vi "LoopVI-V4.vi"() -> ()   [LabVIEW 2013]
uses:
  <vilib>/Utility/file.llb/Read From Spreadsheet File (DBL).vi
panel:
  out "min index(es)":i32
  out "min value":dbl
  out "output array":dbl[](array[numeric])
  out "Collimator afstand":dbl
  out "Spleedbreedte":dbl
  out "Alignment correction":dbl
  out "Background coincidence counts":dbl
  out "Core width":dbl
  out "Fermi Angle":dbl
  out "22na source radius":dbl
  out "Fraction core annihilations":dbl
  out "Minimum summed squared residuals":dbl
  in  "Step size":dbl=1.0 format="%#_13g"
  in  "Begin range":dbl=575.0 format="%#_13g"
  in  "Amount of steps":i32=50
  in  "?":dbl=0.1 format="%#_13g"
  in  "Begin range":dbl=0.5 format="%#_13g"
  in  "Amount of steps":i32=10
  in  "Step size":dbl=0.1 format="%#_13g"
  in  "Begin range":dbl=2.5 format="%#_13g"
  in  "Amount of steps":i32=40
  in  "Step size":dbl=0.1 format="%#_13g"
  in  "Begin range":dbl=1.0 format="%#_13g"
  in  "Amount of steps":dbl=10.0 format="%#_13g"
  in  "Step size":dbl=0.1 format="%#_13g"
  in  "Begin range":dbl=4.0 format="%#_13g"
  in  "Amount of steps":i32=5
  in  "Amount of steps":dbl=4.0 format="%#_13g"
  in  "Step size":dbl=0.1 format="%#_13g"
  in  "Amount of steps":i32=20
  in  "Amount of steps":i32=2
  in  "Begin range":dbl=6.5 format="%#_13g"
  in  "Step size":dbl=0.1 format="%#_13g"
  in  "Begin range":dbl=0.01 format="%#_13g"
  in  "Step size":dbl=0.1 format="%#_13g"
  in  "Begin range":dbl=0.15 format="%#_13g"
  in  "Stop Button":bool
  out "Percentage":dbl format="%#_4f"
  in  "file path (dialog if empty)":path
  in  "Load":bool caption="measurement file\n\n         ??. txt"
  out "free gas model":cluster{"Y":dbl[], "Y":dbl[]}[](graph)
  in  "Fermi angle\n   (mrad)":dbl=7.0
  in  "stop 2":bool
  out "core electrons":cluster{"Y":dbl[], "Y":dbl[]}[](graph)
  in  "core width\n   (mrad)":dbl=5.0
  in  "fraction core\nannihilations":dbl=0.2 min=0.0 max=1.0 step=1e-05
  out "ZICHT  functie":cluster{"Y":dbl[], "Y":dbl[]}[](graph)
  in  "spleetbreedte\n      (mm)":dbl=1.0 min=0.1 max=5.0
  in  "collimator afstand\n       (mm)":dbl=500.0 min=100.0 max=1000.0
  in  "stop 4":bool
  out "XY Graph 4":cluster{ext[], "Array out":ext[]}[](graph)
  in  "alignment correction":dbl min=-10.0 max=10.0 step=0.0001
  in  "background \n coincidence counts":dbl min=0.0 max=100.0
  out "Fermi energy (eV)":dbl format="%#_3g"
  in  "22Na source radius (mm)":dbl=0.1 min=1e-05 max=3.0
  in  "1d - Acar":bool caption="2d - Acar or DB"
  out "2d - Acar 2":bool
  out "2d - Acar 3":bool
  out "2d - Acar 4":bool
  out "XY Graph 5":cluster{ext[], "Array out":ext[]}[](graph)
  out "output cluster 2":cluster{ext[], ext[]}
  out "Sum of squared residuals":dbl
  in  "sigma (mrad) 2":dbl
  # "Step size"
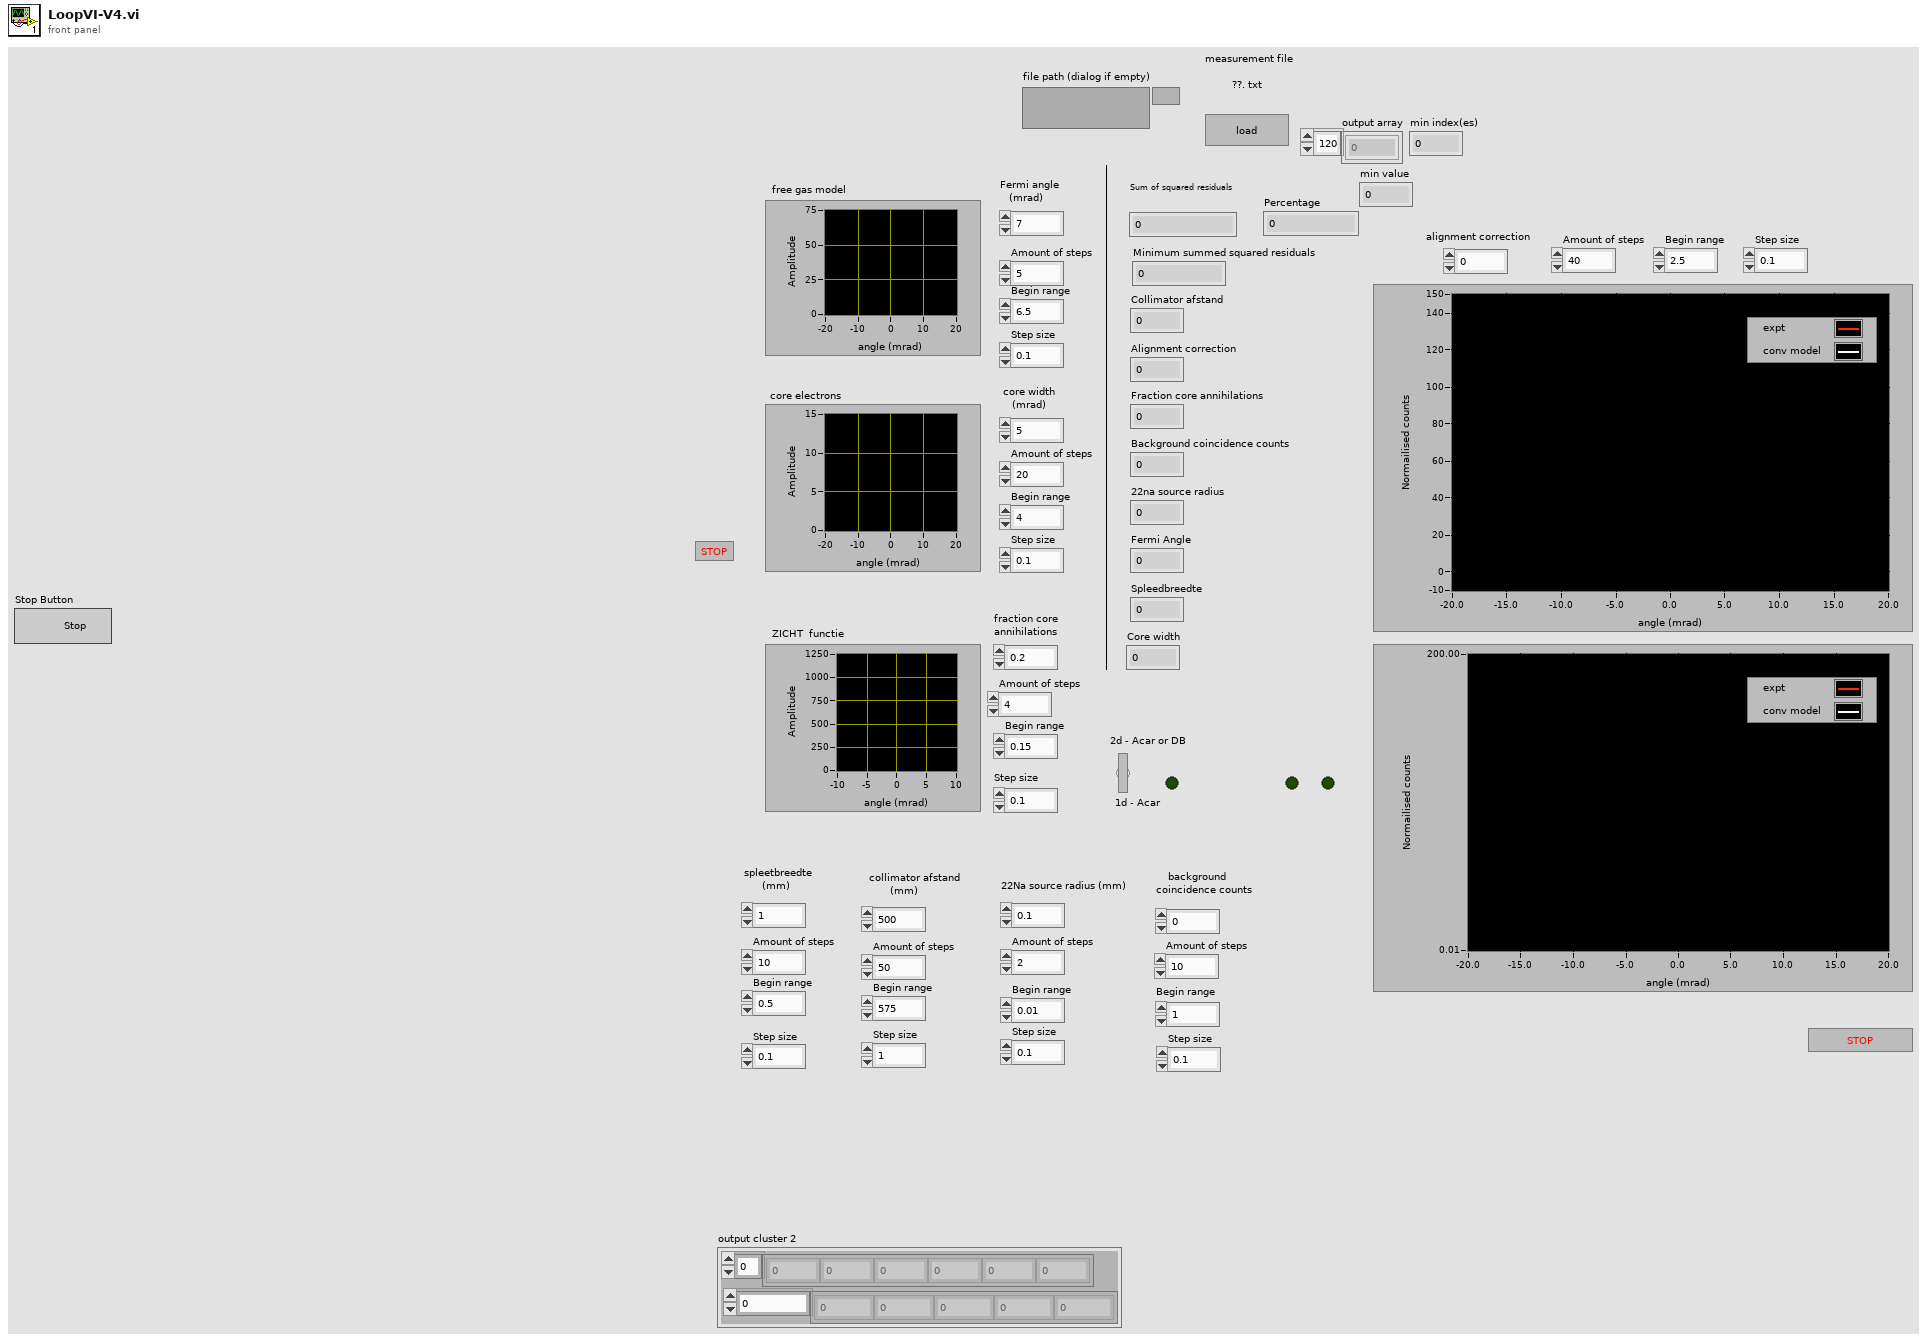
[diagram p1: front panel]
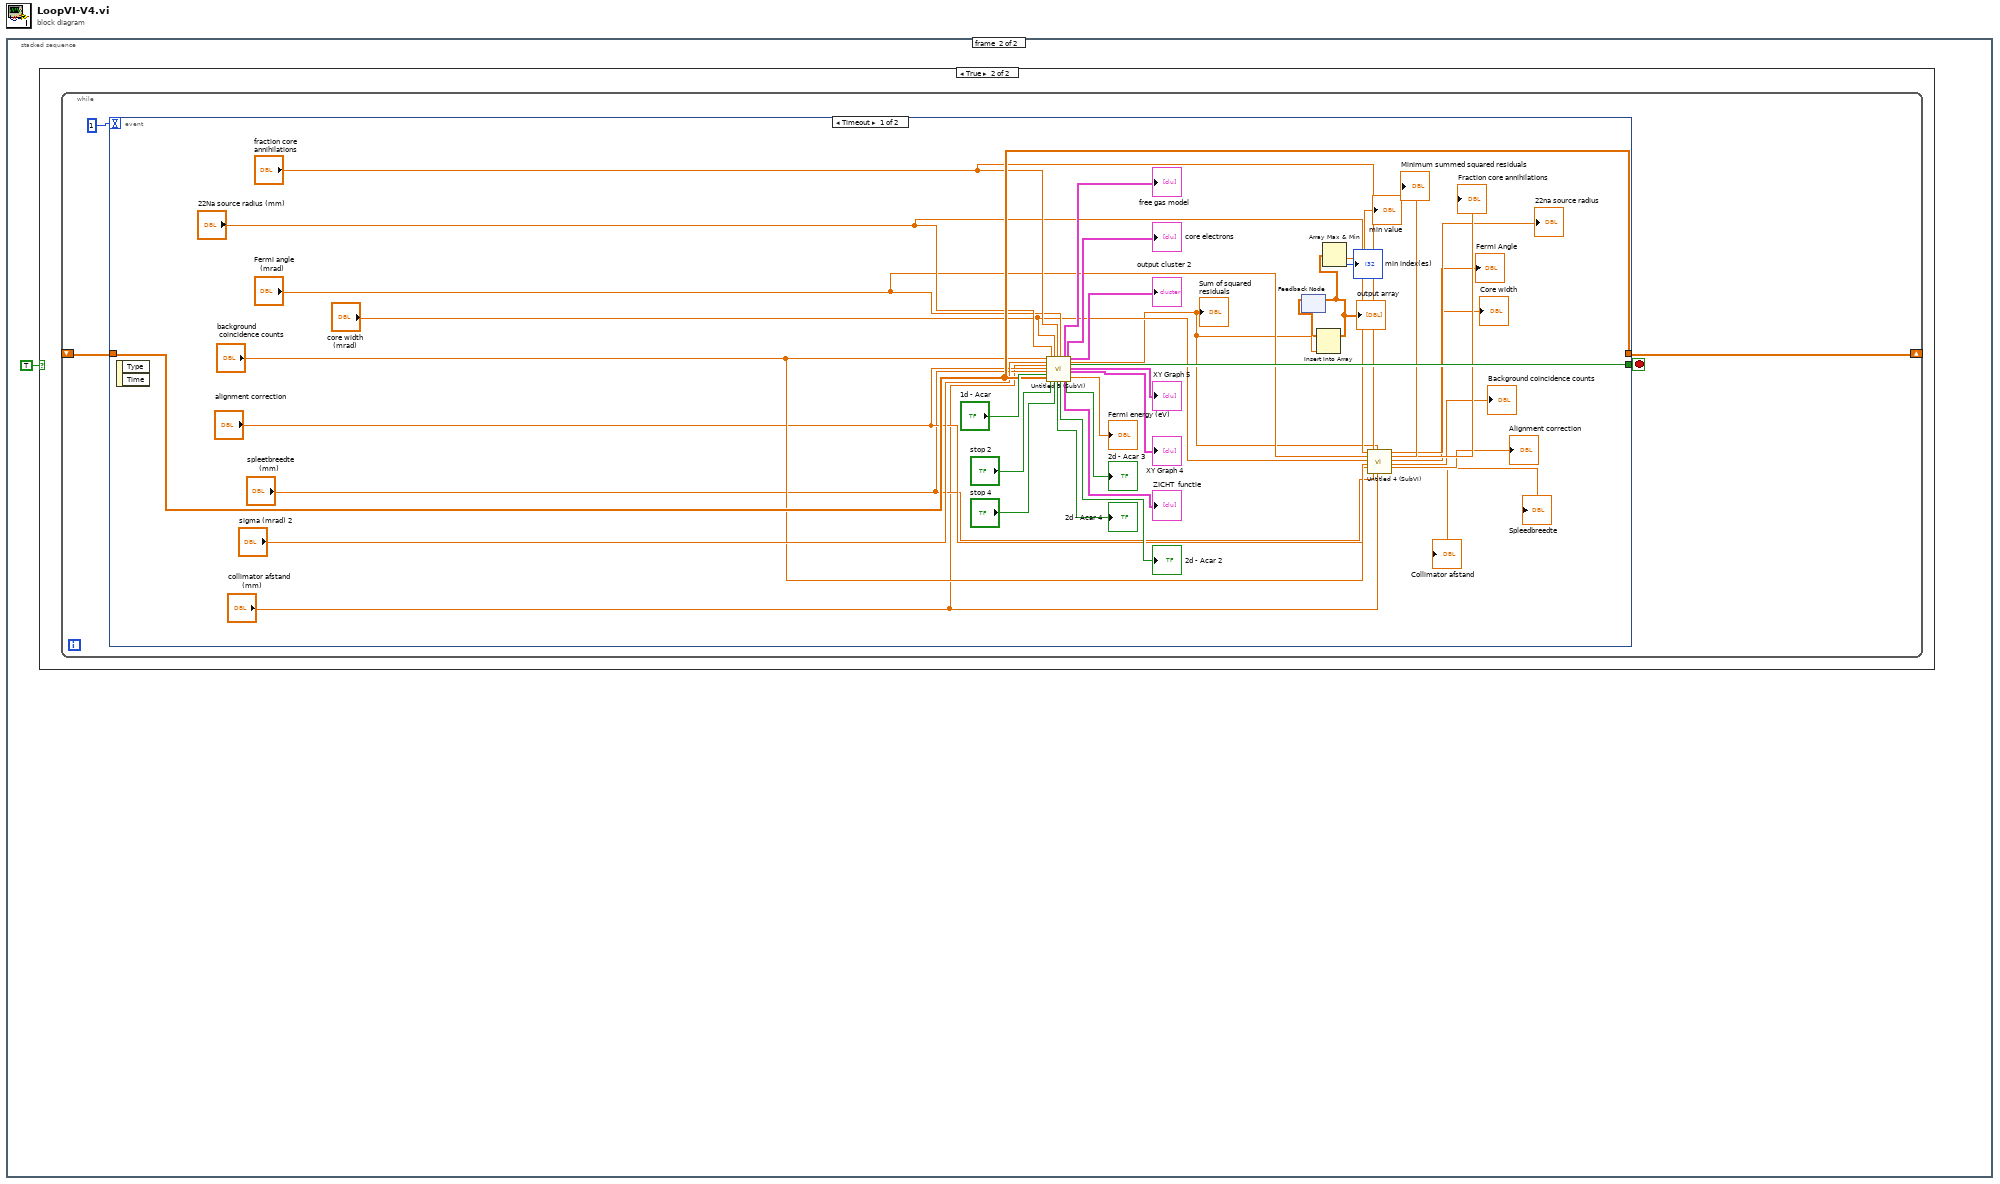
[diagram p0: block diagram]
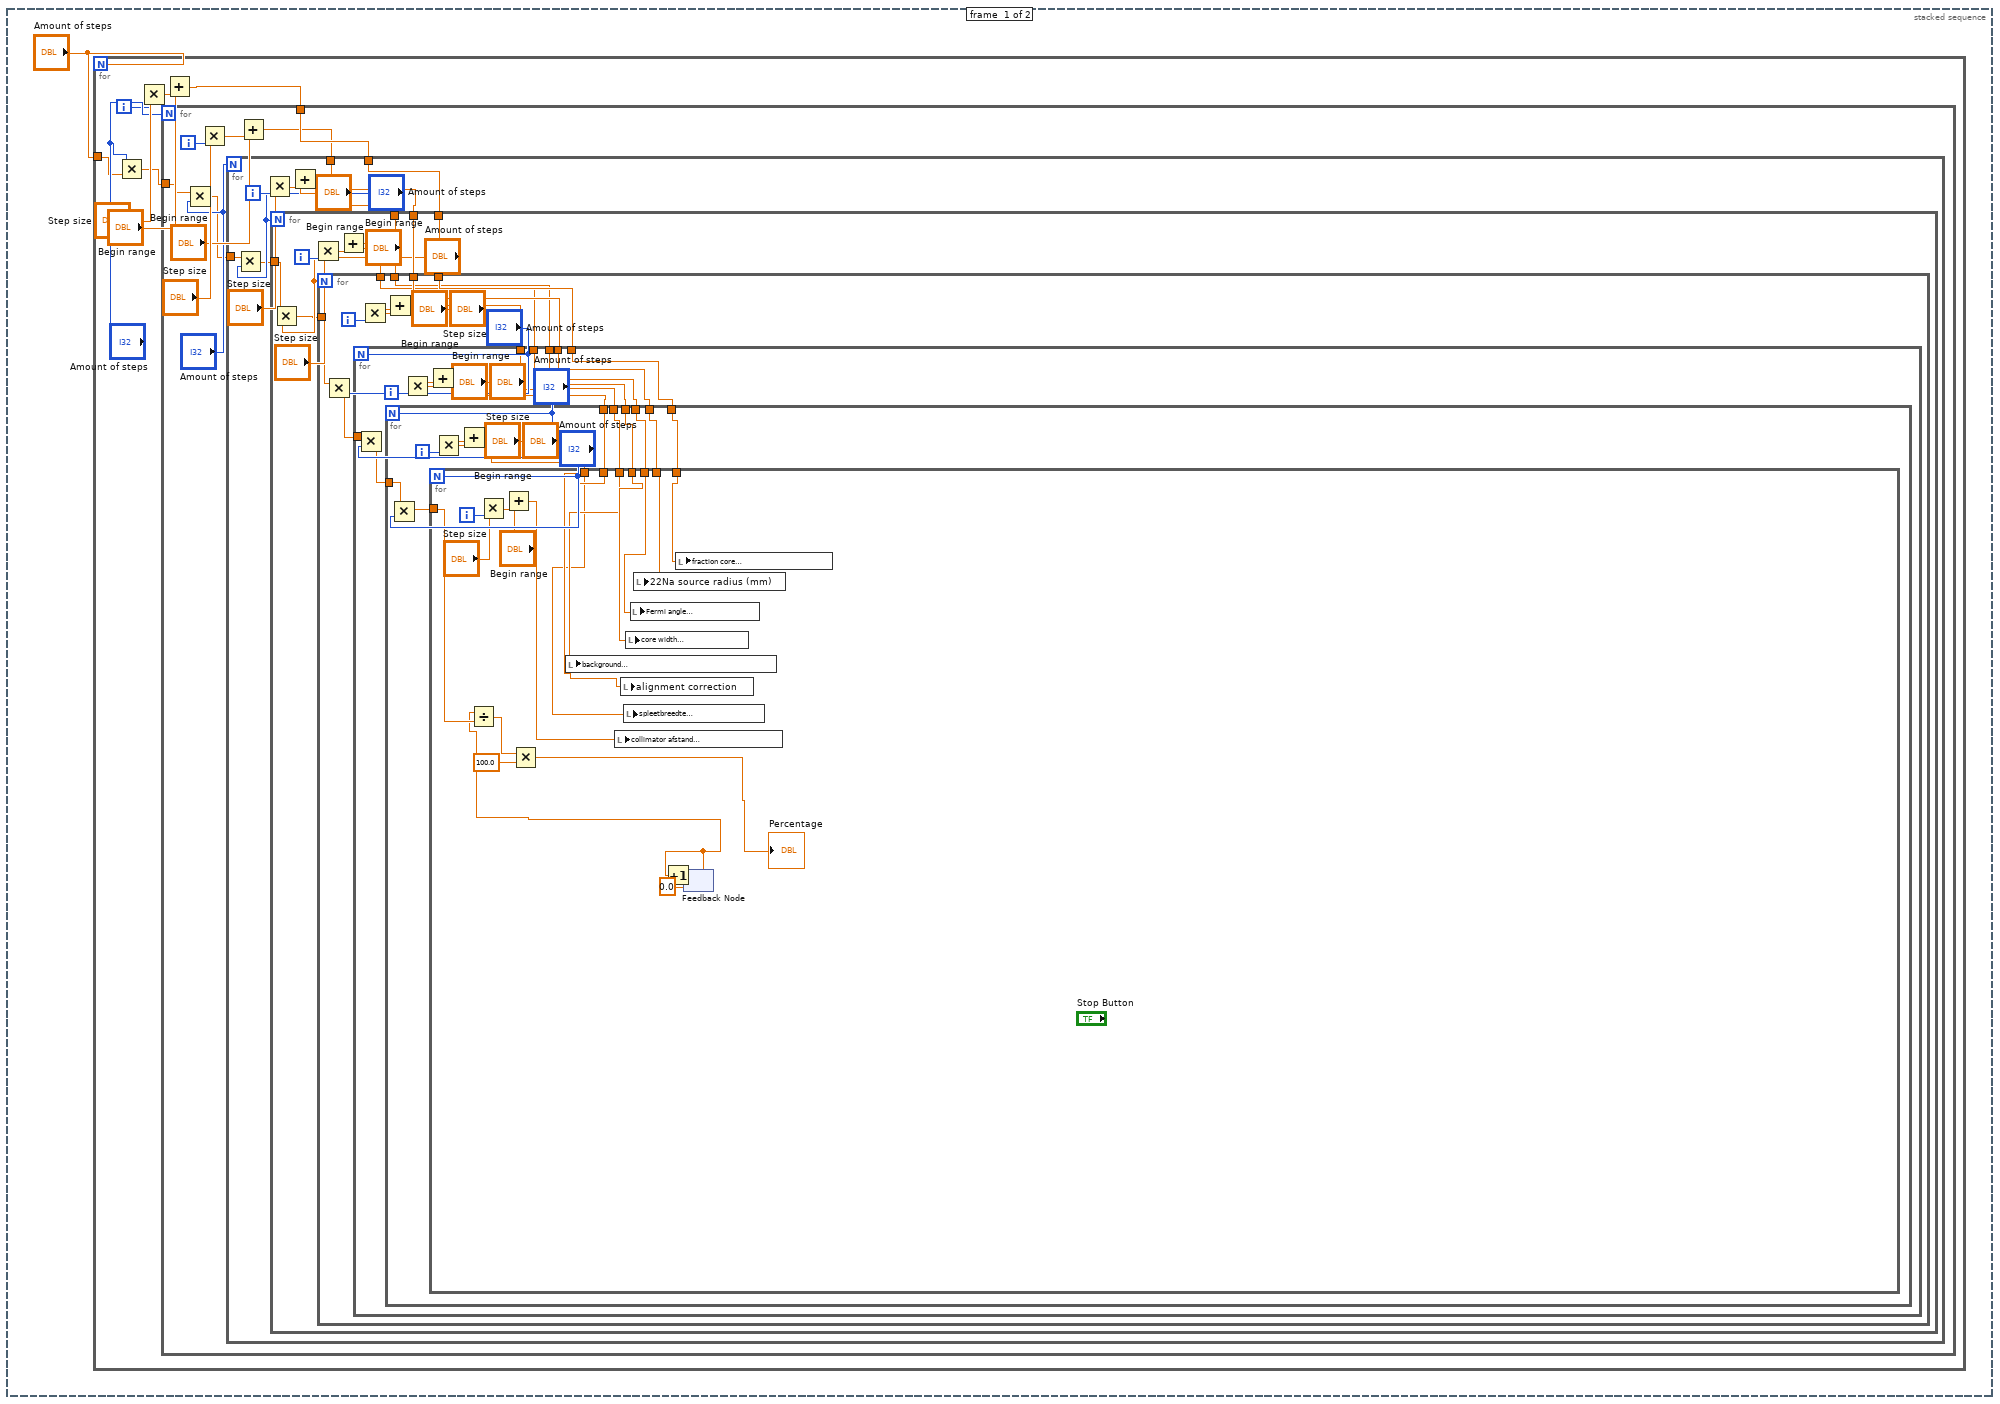
[diagram p2: hidden frame]
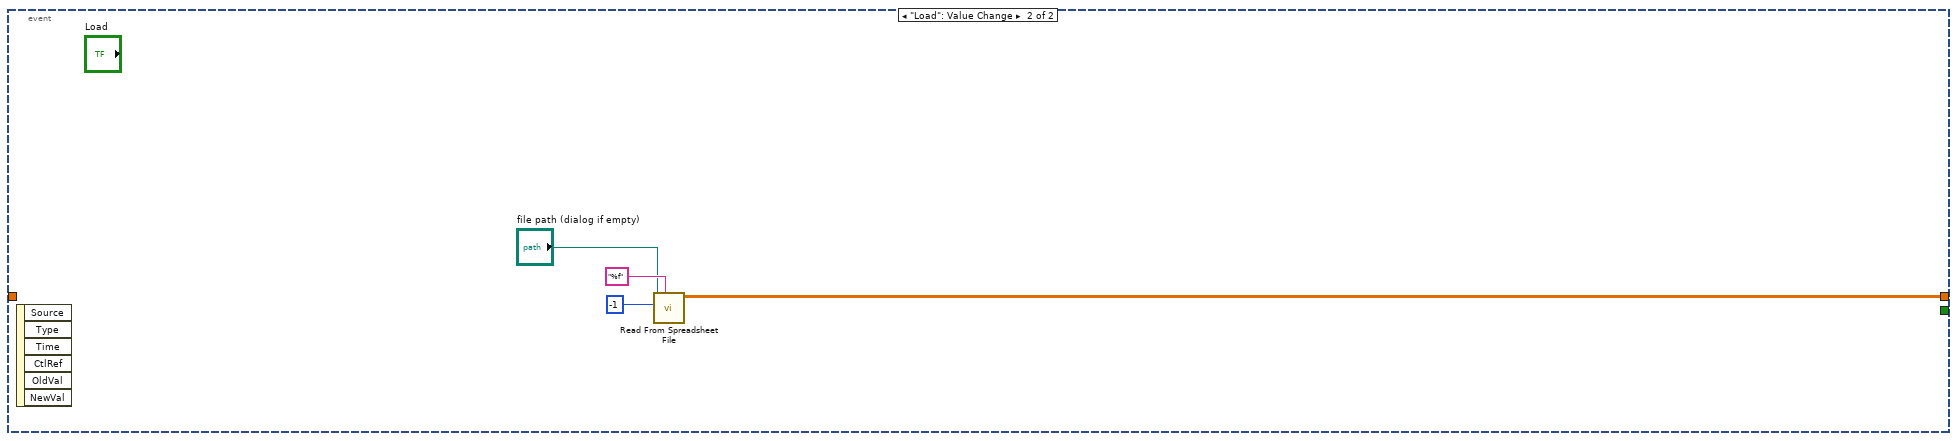
[diagram p4: hidden frame]
diagram:
  n1 = stacked-sequence {
    frame #0 {
      n2 = for {
        N: "Amount of steps" -> [_]
        tunnel: "Amount of steps" -> [w4]
        i -> [w2]
        n3 = Multiply(x="Amount of steps", y=w4) -> (x*y=w3:dbl)
        n4 = Multiply(x="Step size", y=w2) -> (x*y=w8:dbl)
        n5 = Add(x="Begin range", y=w8) -> (x+y=w6:dbl)
        n6 = for {
          N: "Amount of steps" -> [_]
          tunnel: w6 -> [w14]
          tunnel: w3 -> [w12]
          i -> [w18]
          n7 = Multiply(x=w12, y="Amount of steps") -> (x*y=w10:dbl)
          n8 = Multiply(x="Step size", y=w18) -> (x*y=w16:dbl)
          n9 = Add(x="Begin range", y=w16) -> (x+y=w13:dbl)
          n10 = for {
            N: "Amount of steps" -> [_]
            tunnel: w14 -> [w24]
            tunnel: w13 -> [w23]
            tunnel: w10 -> [w21]
            i -> [w28]
            n11 = Multiply(x=w21, y="Amount of steps") -> (x*y=w19:dbl)
            n12 = Multiply(x="Step size", y=w28) -> (x*y=w26:dbl)
            n13 = Add(x="Begin range", y=w26) -> (x+y=w22:dbl)
            n14 = for {
              N: "Amount of steps" -> [_]
              tunnel: w24 -> [w32]
              tunnel: w23 -> [w33]
              tunnel: w22 -> [w34]
              tunnel: w19 -> [w31]
              i -> [w39]
              n15 = Multiply(x=w31, y="Amount of steps") -> (x*y=w29:dbl)
              n16 = Multiply(x="Step size", y=w39) -> (x*y=w37:dbl)
              n17 = Add(x="Begin range", y=w37) -> (x+y=w35:dbl)
              n18 = for {
                N: "Amount of steps" -> [_]
                tunnel: w35 -> [w44]
                tunnel: w34 -> [w45]
                tunnel: w33 -> [w46]
                tunnel: w32 -> [w47]
                tunnel: w29 -> [w42]
                i -> [w51]
                n19 = Multiply(x=w42, y="Amount of steps") -> (x*y=w40:dbl)
                n20 = Multiply(x="Step size", y=w51) -> (x*y=w49:dbl)
                n21 = Add(x="Begin range", y=w49) -> (x+y=w43:dbl)
                n22 = for {
                  N: "Amount of steps" -> [_]
                  tunnel: w47 -> [w60]
                  tunnel: w46 -> [w59]
                  tunnel: w45 -> [w58]
                  tunnel: w44 -> [w57]
                  tunnel: w43 -> [w56]
                  tunnel: w40 -> [w54]
                  i -> [w64]
                  n23 = Multiply(x=w54, y="Amount of steps") -> (x*y=w52:dbl)
                  n24 = Multiply(x="Step size", y=w64) -> (x*y=w62:dbl)
                  n25 = Add(x="Begin range", y=w62) -> (x+y=w55:dbl)
                  n26 = for {
                    N: "Amount of steps" -> [_]
                    tunnel: w60 -> [w73]
                    tunnel: w59 -> [w72]
                    tunnel: w58 -> [w71]
                    tunnel: w57 -> [w70]
                    tunnel: w56 -> [w69]
                    tunnel: w55 -> [w68]
                    tunnel: w52 -> [w67]
                    i -> [w78]
                    n27 = Multiply(x=w67, y="Amount of steps") -> (x*y=w65:dbl)
                    n28 = Multiply(x="?", y=w78) -> (x*y=w76:dbl)
                    n29 = Add(x="Begin range", y=w76) -> (x+y=w74:dbl)
                    n30 = for {
                      N: "Amount of steps" -> [_]
                      tunnel: w74 -> [w87]
                      tunnel: w73 -> [w93]
                      tunnel: w72 -> [w92]
                      tunnel: w71 -> [w91]
                      tunnel: w70 -> [w90]
                      tunnel: w69 -> [w89]
                      tunnel: w68 -> [w88]
                      tunnel: w65 -> [w83]
                      i -> [w97]
                      n31 = Multiply(x="Step size", y=w97) -> (x*y=w95:dbl)
                      n32 = Add(x="Begin range", y=w95) -> (x+y=w86:dbl)
                      n33 = local write "background \n coincidence counts"(w89) -> ()
                      n34 = local write "collimator afstand\n       (mm)"(w86) -> ()
                      n35 = local write "alignment correction"(w88) -> ()
                      n36 = local write "spleetbreedte\n      (mm)"(w87) -> ()
                      n37 = local write "core width\n   (mrad)"(w90) -> ()
                      n38 = local write "Fermi angle\n   (mrad)"(w91) -> ()
                      n39 = local write "22Na source radius (mm)"(w92) -> ()
                      n40 = local write "fraction core\nannihilations"(w93) -> ()
                      n41 = feedback #1(0.0) -> (w82:dbl)
                      n42 = Divide(x=w82, y=w83) -> (x/y=w81:dbl)
                      n43 = Multiply(x=w81, y=100.0) -> (x*y=→"Percentage":dbl)
                      n44 = Increment(x=w82) -> (x+1=w85:dbl)
                      n45 = feedback-in #1(w85) -> ()
                    }
                  }
                }
              }
            }
          }
        }
      }
    }
    frame #1 {
      n46 = case shown="True" TRUE {
        frame False {
        }
        frame True {
          n47 = while {
            shift-right: [w100] -> _
            shift-left: _ -> [w99]
            stop <- w102 stop-if-true
            n48 = event shown="[0] Timeout" {
              selector: _ -> [_ _]
              dyn-events: _ -> [_ _]
              timeout: 1 -> [_ _]
              tunnel: [w140 _] -> w102
              tunnel: [w138 w143] -> w100
              tunnel: w99 -> [w138 _]
              event Timeout {
                n49 = event-data() -> ()  [unwired: 1 in, 2 out]
                n50 = call "Untitled 9 (SubVI).vi"("background \n coincidence counts"="background \n coincidence counts", "sigma (mrad) in"="sigma (mrad) 2", "collimator afstand\n       (mm)"="collimator afstand\n       (mm)", "alignment correction"="alignment correction", "spleetbreedte\n      (mm)"="spleetbreedte\n      (mm)", "1d - Acar"="1d - Acar", "all rows"=w138, "22Na source radius (mm)"="22Na source radius (mm)", "stop in"="stop 2", "core width\n   (mrad)"="core width\n   (mrad)", "stop 4"="stop 4", "fraction core\nannihilations"="fraction core\nannihilations", "Fermi angle\n   (mrad)"="Fermi angle\n   (mrad)") -> ("2d - Acar 4"=→"2d - Acar 4":bool, "2d - Acar 2"=→"2d - Acar 2":bool, "free gas model"=→"free gas model":cluster{"Y":dbl[], "Y":dbl[]}[], "ZICHT  functie"=→"ZICHT  functie":cluster{"Y":dbl[], "Y":dbl[]}[], "core electrons"=→"core electrons":cluster{"Y":dbl[], "Y":dbl[]}[], "2d - Acar 3"=→"2d - Acar 3":bool, "output cluster 2"=→"output cluster 2":cluster{ext[], ext[]}, "Sum of squared residuals"=w107:dbl, "stop 3"=w140:bool, "XY Graph 5"=→"XY Graph 5":cluster{ext[], "Array out":ext[]}[], "XY Graph 4"=→"XY Graph 4":cluster{ext[], "Array out":ext[]}[], "Fermi energy (eV)"=→"Fermi energy (eV)":dbl)  [unwired: 2 in, 1 out]
                "Sum of squared residuals" <- w107
                n51 = feedback #2() -> (w106:dbl[])  [unwired: 1 in]
                n52 = Insert Into Array(array=w106, new element=w107) -> (w105:dbl[])  [unwired: 1 in]
                "output array" <- w105
                n53 = feedback-in #2(w105) -> ()
                n54 = Array Max & Min(array=w105) -> (min value=→"min value":dbl, min index (indices)=→"min index(es)":i32)  [unwired: 2 out]
                n55 = call "Untitled 4 (SubVI).vi"("x 19"="22Na source radius (mm)", "x 18"="Fermi angle\n   (mrad)", "x 17"="core width\n   (mrad)", "x 16"="background \n coincidence counts", "x 15"="alignment correction", "x 20"="fraction core\nannihilations", "x 14"="spleetbreedte\n      (mm)", "x 4"=w107, "x 13"="collimator afstand\n       (mm)") -> ("x 3"=→"Minimum summed squared residuals":dbl, "x 12"=→"Collimator afstand":dbl, "x 5"=→"Fraction core annihilations":dbl, "x 11"=→"Spleedbreedte":dbl, "x 6"=→"22na source radius":dbl, "x 7"=→"Fermi Angle":dbl, "x 8"=→"Core width":dbl, "x 9"=→"Background coincidence counts":dbl, "x 10"=→"Alignment correction":dbl)  [unwired: 2 in]
              }
              event "Load": Value Change {
                n56 = event-data() -> ()  [unwired: 1 in, 6 out]
                n57 = call-poly <vilib>:"Read From Spreadsheet File.vi"("format (%.3f)"="%f", "number of rows (all:-1)"=-1, "file path (dialog if empty)"="file path (dialog if empty)") -> ("all rows"=w143:ext[][])  [unwired: 4 in, 4 out]
              }
            }
          }
        }
      }
    }
  }
